vi "COMMAND_GoToRelativePosition.vi"(8 "error in (no error)":errorcluster, 10 "target  position":refnum<class "SpaceVector.lvclass">, 11 "MH100301DMC in":refnum<class "StageMH100301DMC.lvclass">) -> (0 "error out":errorcluster, 3 "MH100301DMC out":refnum<class "StageMH100301DMC.lvclass">)   [LabVIEW 2010, in "StageMH100301DMC.lvclass"]
uses:
  StageMH100301DMC.lvclass
  common/classes/SpaceVector/SpaceVector/SpaceVector.lvclass
  StageMH100301DMC.lvclass/StageMH100301DMC.ctl
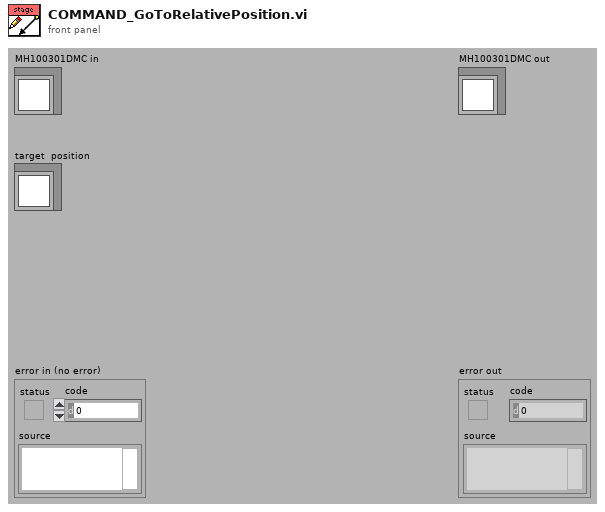
[diagram p1: front panel]
types:
  T1 = typedef "space_vector_array.ctl" = dbl[unit][]
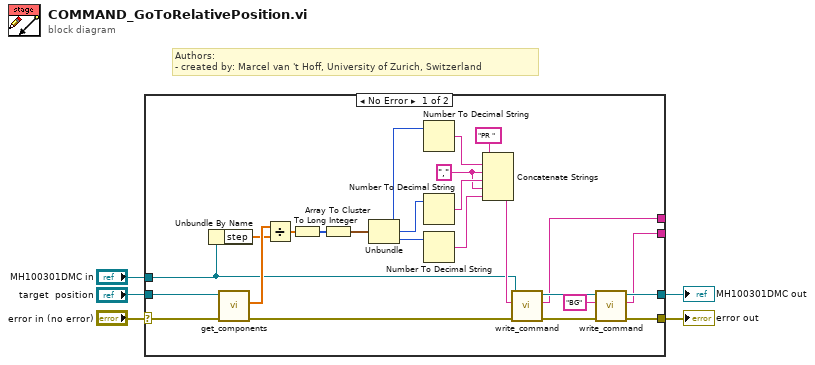
[diagram p0: block diagram]
diagram:
  # "Authors: \n- created by: Marcel van 't Hoff, University of Zurich, Switzerland"
  n1 = case shown="No Error" "error in (no error)" {
    selector: "error in (no error)" -> [w29 w32]
    tunnel: [w11 w32] -> w4
    tunnel: [w13 w31] -> w2
    tunnel: "MH100301DMC in" -> [w6 w31]
    tunnel: "target  position" -> [w30 _]
    tunnel: [w9 _] -> _
    tunnel: [w7 _] -> _
    frame No Error {
      w15 = ","
      n2 = Unbundle By Name(w6) -> ("step"=w8:dbl[unit][])
      n3 = call "get_components.vi"("error in (no error)"=w29, "SpaceVector in"=w30) -> ("error out"=w24:errorcluster, "x/y/z"=w23:T1)  [unwired: 8 out]
      n4 = Divide(x=w23, y=w8) -> (x/y=w21:dbl[])
      n5 = To Long Integer(number=w21) -> (32bit integer=w20:i32[])
      n6 = Array To Cluster(array=w20) -> (cluster=w22:cluster{"[0]":i32, "[1]":i32, "[2]":i32})
      n7 = Unbundle(w22) -> ("[0]"=w19:i32, "[1]"=w18:i32, "[2]"=w17:i32)
      n8 = Number To Decimal String(number=w19) -> (decimal integer string=w27:string)  [unwired: 1 in]
      n9 = Number To Decimal String(number=w18) -> (decimal integer string=w16:string)  [unwired: 1 in]
      n10 = Number To Decimal String(number=w17) -> (decimal integer string=w26:string)  [unwired: 1 in]
      n11 = Concatenate Strings("PR ", w27, w15, w16, w15, w26) -> (w25:string)
      n12 = call-dynamic "write_command.vi"("error in (no error)"=w24, "command (without terminating \"\\n\")"=w25, "MH100301DMC in"=w6) -> ("error out"=w12:errorcluster, "response out"=w7:string, "MH100301DMC out"=w14:refnum<class "StageMH100301DMC.lvclass">)  [unwired: 1 in, 5 out]
      n13 = call-dynamic "write_command.vi"("error in (no error)"=w12, "command (without terminating \"\\n\")"="BG" ("command (without terminating \"\\n\")"), "MH100301DMC in"=w14) -> ("error out"=w11:errorcluster, "response out"=w9:string, "MH100301DMC out"=w13:refnum<class "StageMH100301DMC.lvclass">)  [unwired: 1 in, 5 out]
    }
    frame Error {
    }
  }
  "error out" <- w4
  "MH100301DMC out" <- w2
